vi "Plug_in_for_Samantha.vi"() -> (5 "Plug in titles":string[](array[string]), 7 "Plug in values":string[](array[string]))   [LabVIEW 2010]
uses:
  Globals/Meas_global.vi
  Globals/Constants_global.vi
  Globals/Plug_in_data_global.vi
panel:
  in  "Boundary layer type":string
  in  "Obstruction type":string
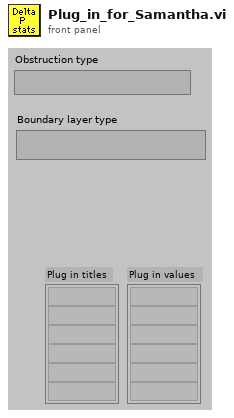
[diagram p1: front panel]
types:
  T1 = typedef "Analysis_info_cluster.ctl" = cluster{"Colour":u32, "Inst type":T2, "Inst name":string, "Symbol":string, "Code name":string, "Extra Info":string, "Inst Array":T3, "Index":i32, "Voltage Index":i32, "Extra Titles":string[], "Extra Values":string[]}
  T2 = typedef "Inst_type.ctl" = enum16{"Propeller anemometer", "Raw voltage", "Pressure Transducer", "Pitot-static tube", "Preston tube", "Hot wire", "Cross wire 1", "Cross wire 2", "Generic Linear", "Generic Polynomial", "Generic BackPoly", "Fast FID", "Thermocouple", "Cold wire", "Pulsed Wire", "LDA Vel", "LDA Tran time", "LDA Arr time"}
  T3 = typedef "Instrument_Array.ctl" = enum16{"PWA", "LDA", "Analogue"}
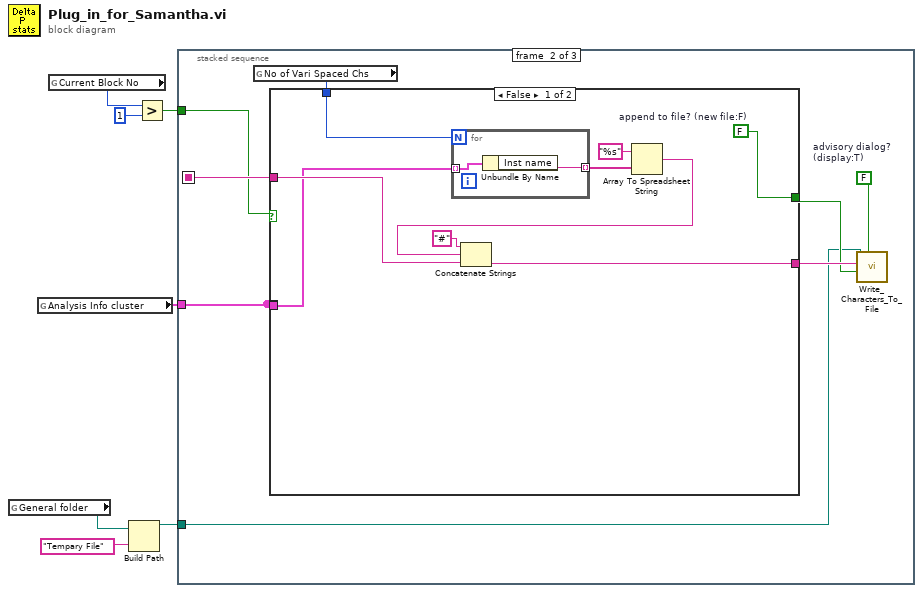
[diagram p0: block diagram]
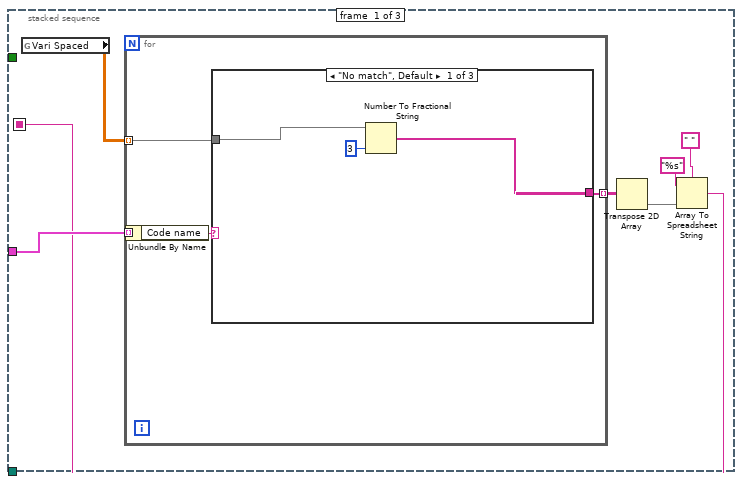
[diagram p2: hidden frame]
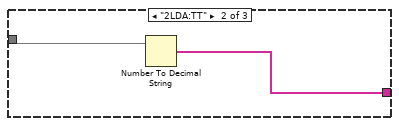
[diagram p3: hidden frame]
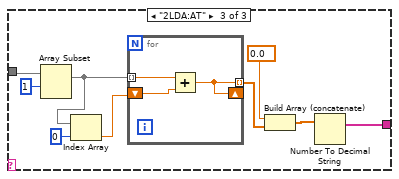
[diagram p4: hidden frame]
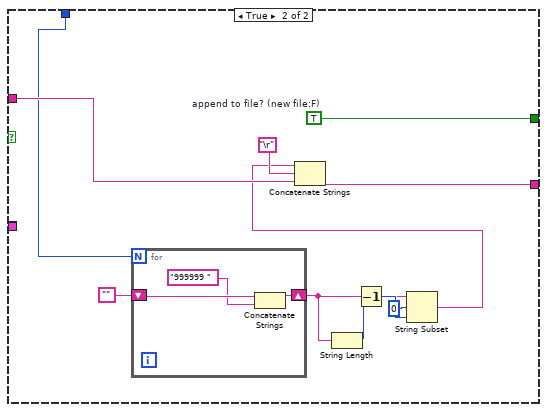
[diagram p5: hidden frame]
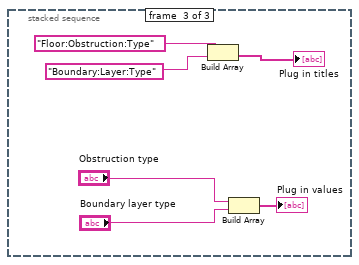
[diagram p6: hidden frame]
diagram:
  n1 = global read "Constants_global.vi" "General folder"() -> (w3:path)
  n2 = global read "Meas_global.vi" "Analysis Info cluster"() -> (w4:T1[])
  n3 = global read "Meas_global.vi" "Current Block No"() -> (w6:i32)
  n4 = Build Path(base path=w3, name or relative path="Tempary File") -> (appended path=w1:path)
  n5 = Greater?(x=w6, y=1) -> (0:w5:bool)
  n6 = stacked-sequence {
    seq-local: [w8 _ _] -> [_ w42 _]
    tunnel: w5 -> [_ w40 _]
    tunnel: w4 -> [w13 w38 _]
    tunnel: w1 -> [_ w37 _]
    frame #0 {
      n7 = global read "Plug_in_data_global.vi" "Vari Spaced"() -> (w14:dbl[][])
      n8 = for {
        tunnel: w13 -> [w18] mode=indexing
        tunnel: w14 -> [w16] mode=indexing
        tunnel: [w15] -> w12 mode=indexing
        n9 = Unbundle By Name(w18) -> ("Code name"=w17:string)
        n10 = case shown="\"No match\", Default" w17 {
          tunnel: w16 -> [w21 w23 w32]
          tunnel: [w20 w22 w24] -> w15
          frame "No match", Default {
            n11 = Number To Fractional String(number=w21, precision (6)=i16 3) -> (F-format string=w20:string[])  [unwired: 2 in]
          }
          frame "2LDA:TT" {
            n12 = Number To Decimal String(number=w23) -> (decimal integer string=w22:string[])  [unwired: 1 in]
          }
          frame "2LDA:AT" {
            n13 = Array Subset(array=w32, index=1) -> (w28:dbl[])  [unwired: 1 in]
            n14 = Index Array(array=w28, index=0 ("Index")) -> (element=w26:dbl)
            n15 = for {
              shift-right: [w33] -> _
              shift-left: w26 -> [w35]
              tunnel: w28 -> [w34] mode=indexing
              tunnel: [w33] -> w30 mode=indexing
              n16 = Add(x=w34, y=w35) -> (x+y=w33:dbl)
            }
            n17 = Build Array (concatenate)(0.0, w30) -> (w25:dbl[])
            n18 = Number To Decimal String(number=w25) -> (decimal integer string=w24:string[])  [unwired: 1 in]
          }
        }
      }
      n19 = Transpose 2D Array(2D array=w12) -> (transposed array=w9:string[][])
      n20 = Array To Spreadsheet String(delimiter (Tab)=" ", array=w9, 3:"%s" ("format string")) -> (spreadsheet string=w8:string)
    }
    frame #1 {
      w39 = FALSE  # advisory dialog? (display:T)
      n21 = global read "Meas_global.vi" "No of Vari Spaced Chs"() -> (w36:i32)
      n22 = case shown="False" w40 {
        tunnel: [w52 w65] -> w43
        tunnel: w42 -> [w51 w64]
        tunnel: [w50 w63] -> w41
        tunnel: w38 -> [_ _]
        tunnel: w38 -> [w47 _]
        tunnel: w36 -> [w44 w55]
        frame False {
          w50 = FALSE  # append to file? (new file:F)
          n23 = for {
            N: w44 -> [_]
            tunnel: w47 -> [w54] mode=indexing
            tunnel: [w53] -> w48 mode=indexing
            n24 = Unbundle By Name(w54) -> ("Inst name"=w53:string)
          }
          n25 = Array To Spreadsheet String(array=w48, 3:"%s" ("format string")) -> (spreadsheet string=w46:string)  [unwired: 1 in]
          n26 = Concatenate Strings("#" ("Substring"), w46, w51) -> (w52:string)
        }
        frame True {
          w63 = TRUE  # append to file? (new file:F)
          n27 = for {
            N: w55 -> [_]
            shift-right: [w66] -> w57
            shift-left: "" -> [w68]
            n28 = Concatenate Strings(w68, "999999 ") -> (w66:string)
          }
          n29 = String Length(string=w57) -> (length=w59:i32)
          n30 = Decrement(x=w59) -> (x-1=w58:i32)
          n31 = String Subset(string=w57, offset (0)=0, length (rest)=w58) -> (substring=w56:string)
          n32 = Concatenate Strings(w56, "\r", w64) -> (w65:string)
        }
      }
      n33 = call "Write_Characters_To_File.vi"("file path (dialog if empty)"=w37, "advisory dialog? (display:T)"=w39, "character string"=w43, "append to file? (new file:F)"=w41) -> ()  [unwired: 4 in, 1 out]
    }
    frame #2 {
      n34 = Build Array("Floor:Obstruction:Type" ("Obstruction type"), "Boundary:Layer:Type" ("Obstruction type")) -> (→"Plug in titles":string[])
      n35 = Build Array("Obstruction type", "Boundary layer type") -> (→"Plug in values":string[])
    }
  }
